vi "ProdaNG.Tree.Selection.GetTS.vi"(7 "TestStepsTree":refnum<vi>, 8 "error in (no error)":errorcluster) -> (0 "error out":errorcluster, 2 "LastTS":T1)   [LabVIEW 2016]
uses:
  ProdaNG.Tree.Fglb.Data.ctl
  ProdaNG.Tree.Fglb.Element.ctl
  ProdaNG.Tree.Fglb.Action.ctl
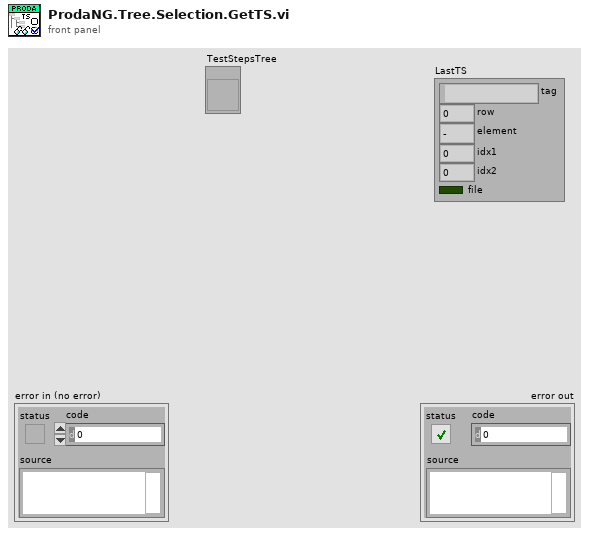
[diagram p1: front panel]
types:
  T1 = typedef "ProdaNG.Tree.Fglb.Data.ctl" = cluster{"tag":string, "row":i32, "element":T2, "idx1":i32, "idx2":i32, "file":bool}
  T2 = typedef "ProdaNG.Tree.Fglb.Element.ctl" = enum16{"-", "PP", "TS", "TP", "TV"}
  T3 = typedef "ProdaNG.Tree.Fglb.Action.ctl" = enum16{"init", "add", "get by row", "get by tag", "get by idx"}
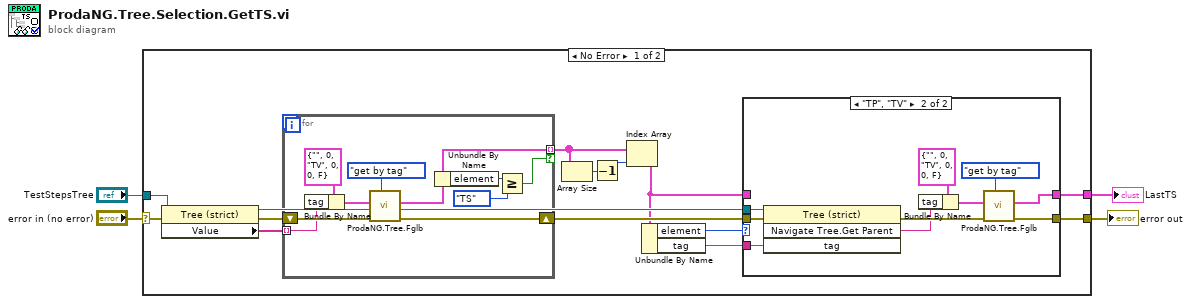
[diagram p0: block diagram]
diagram:
  n1 = case shown="No Error" "error in (no error)" {
    selector: "error in (no error)" -> [w18 w40]
    tunnel: "TestStepsTree" -> [w16 _]
    tunnel: [w9 w40] -> w4
    tunnel: [w8 _] -> w1
    frame No Error {
      n2 = property on="Property Node" class="Tree (strict)"(reference=w16, error in=w18) -> (reference out=w10:refnum<vi>, error out=w17:errorcluster, "Value"=w15:string[])
      n3 = for {
        tunnel: w15 -> [w32] mode=indexing
        shift-right: [w35] -> w11
        shift-left: w17 -> [w36]
        tunnel: [w33] -> w12 mode=indexing if=w30
        n4 = Bundle By Name(cluster=T1 {"tag"="", "row"=0, "element"=enum."TV", "idx1"=0, "idx2"=0, "file"=FALSE} ("entry in"), "tag"=w32) -> (w37:T1)
        n5 = call "ProdaNG.Tree.Fglb.vi"("Action (add)"=ProdaNG.Tree.Fglb.Action."get by tag", "error in"=w36, "entry in"=w37) -> ("error out"=w35:errorcluster, "found entry"=w33:T1)  [unwired: 6 in, 1 out]
        n6 = Unbundle By Name(w33) -> ("element"=w34:T2)
        n7 = Greater Or Equal?(x=w34, y=ProdaNG.Tree.Fglb.Element."TS") -> (x >= y?=w30:bool)
      }
      n8 = Array Size(array=w12) -> (size(s)=w14:i32)
      n9 = Decrement(x=w14) -> (x-1=w13:i32)
      n10 = Index Array(array=w12, index=w13) -> (element=w5:T1)
      n11 = Unbundle By Name(w5) -> ("element"=w6:T2, "tag"=w7:string)
      n12 = case shown="\"TP\", \"TV\"" w6 {
        tunnel: w11 -> [w19 w29]
        tunnel: w10 -> [_ w28]
        tunnel: [w19 w27] -> w9
        tunnel: [w20 w22] -> w8
        tunnel: w7 -> [_ w21]
        tunnel: w5 -> [w20 _]
        frame Default {
        }
        frame "TP", "TV" {
          n13 = invoke class="Tree (strict)" method="Navigate Tree.Get Parent"(reference=w28, error in=w29, "tag"=w21) -> (error out=w27:errorcluster, "Navigate Tree:Get Parent"=w23:string)  [unwired: 1 in, 2 out]
          n14 = Bundle By Name(cluster=T1 {"tag"="", "row"=0, "element"=enum."TV", "idx1"=0, "idx2"=0, "file"=FALSE} ("entry in"), "tag"=w23) -> (w26:T1)
          n15 = call "ProdaNG.Tree.Fglb.vi"("Action (add)"=ProdaNG.Tree.Fglb.Action."get by tag", "entry in"=w26) -> ("found entry"=w22:T1)  [unwired: 7 in, 2 out]
        }
      }
    }
    frame Error {
    }
  }
  "error out" <- w4
  "LastTS" <- w1
